vi "ingest.trigger_file_ingest-existing_dataset.vi"(7 "Timestamp Metadata":refnum<class "timestampMetadata.lvclass">, 8 "error in":errorcluster, 9 "Dataset RID":string, 10 "S3 Path to File":string, 11 "Nominal Client in":refnum<class "Nominal Client.lvclass">) -> (0 "error out":errorcluster, 2 "Information":T1, 3 "Nominal Client out":refnum<class "Nominal Client.lvclass">, 4 "Response":string)   [LabVIEW 2020, in "Nominal Client.lvclass"]
doc: "Triggers an ingest job of a new file, allowing either creating a new dataset or uploading to an existing one."
uses:
  Nominal Client.lvclass
  4b965f09-dc68-4d5e-a5c1-32d476accfd4.vi
  <vilib>/JDP Science/JSONtext/JSON text to Variant.vi
  <vilib>/JDP Science/JSONtext/LVClass Serializer/JSONtext LVClass Serializer.lvclass
  Nominal Client.lvclass/Nominal Client.ctl
  timestampMetadata/timestampMetadata.lvclass
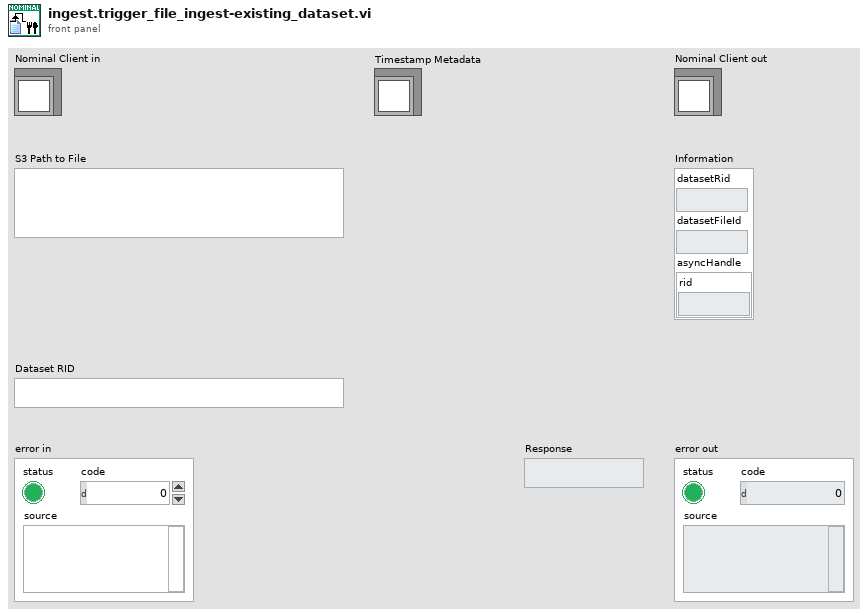
[diagram p1: front panel]
types:
  T1 = cluster{"datasetRid":string, "datasetFileId":string, "asyncHandle":cluster{"rid":string}}
  T2 = cluster{"type":string, "s3":cluster{"path":string}}
  T3 = cluster{"existing_dataset":cluster{"dataset_rid":string}}
  T4 = cluster{"source":cluster{"type":string, "s3":cluster{"path":string}}, "destination":cluster{"existing_dataset":cluster{"dataset_rid":string}}, "sourceMetadata":cluster{"timestampMetadata":string}}
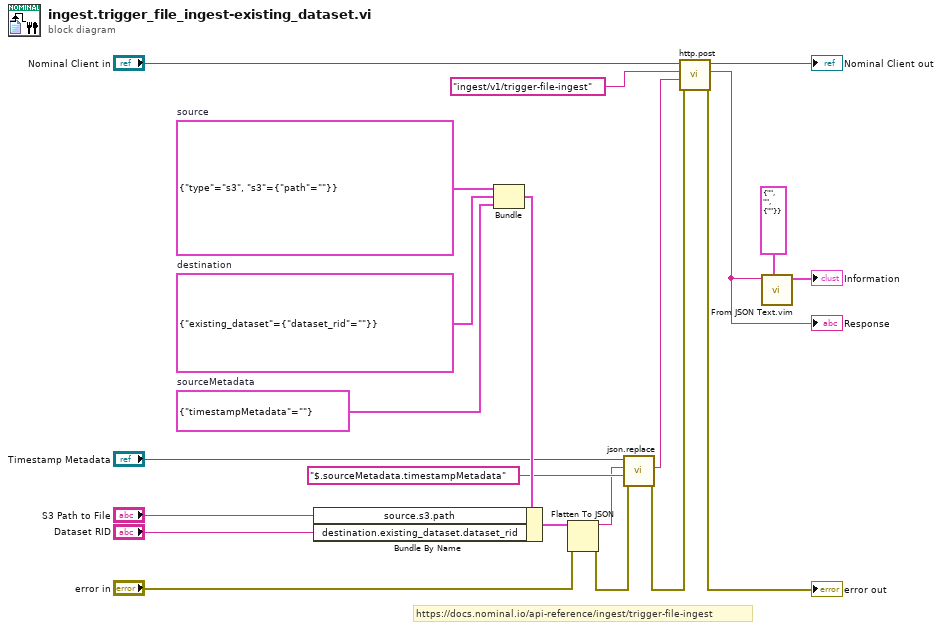
[diagram p0: block diagram]
diagram:
  w15 = T2 {"type"="s3", "s3"={"path"=""}}  # source
  w16 = cluster{"timestampMetadata":string} {"timestampMetadata"=""}  # sourceMetadata
  w17 = T3 {"existing_dataset"={"dataset_rid"=""}}  # destination
  # "https://docs.nominal.io/api-reference/ingest/trigger-file-ingest"
  n1 = Bundle("source"=w15, "destination"=w17, "sourceMetadata"=w16) -> (w7:T4)  [unwired: 1 in]
  n2 = Bundle By Name(cluster=w7, "source.s3.path"="S3 Path to File", "destination.existing_dataset.dataset_rid"="Dataset RID") -> (w14:T4)
  n3 = Flatten To JSON(anything=w14, error in (no error)="error in") -> (JSON string=w2:string, 11:w4:errorcluster)  [unwired: 1 in]
  n4 = call "json.replace.vi"("error in"=w4, "Object To Update"="$.sourceMetadata.timestampMetadata" ("Object Name"), "JSON in"=w2, "timestampMetadata in"="Timestamp Metadata") -> ("error out"=w3:errorcluster, "JSON out"=w1:string)  [unwired: 5 in, 1 out]
  n5 = call "http.post.vi"("error in"=w3, "Request body"=w1, "Path"="ingest/v1/trigger-file-ingest", "Nominal Client in"="Nominal Client in") -> ("error out"=→"error out":errorcluster, "Response"=w8:string, "Nominal Client out"=→"Nominal Client out":refnum<class "Nominal Client.lvclass">)  [unwired: 4 in, 1 out]
  "Response" <- w8
  n6 = call "From JSON Text.vim"("Data Type and Default Value"=T1 {"datasetRid"="", "datasetFileId"="", "asyncHandle"={"rid"=""}} ("Information"), "JSON"=w8) -> ("Data out"=→"Information":T1)  [unwired: 8 in, 1 out]
